vi "continue frame scan.vi"(7 "Max queue size":i32, 8 "Error in":errorcluster, 10 "Scan Status in":enum16{"Start", "Continue Scan", "Finish Scan"}(ring), 11 "Scan Type [in":T1) -> (0 "Error Out":errorcluster)   [LabVIEW 2018]
uses:
  Controls/ScanType.ctl
  Controls/QueueNames.ctl
  Controls/MessagePacket.ctl
  Controls/Queue Manager Actions.ctl
  Controls/FGV Actions.ctl
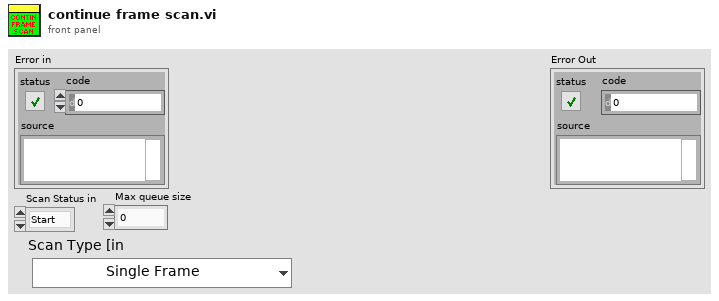
[diagram p1: front panel]
types:
  T1 = typedef "ScanType.ctl" = enum16{"Single Frame", "Continuous Frame", "ROI Line", "Vibratome", "Mosaic", "Mosaic + Slice"}
  T2 = typedef "Queue Manager Actions.ctl" = enum16{"Init", "Enqueue", "Enqueue All", "Preview Queue", "Dequeue", "Get Status", "Flush Queue", "Flush All Queues", "Release All Queues", "Release Queue", "Enqueue at Opposite End"}
  T3 = typedef "MessagePacket.ctl" = cluster{"Message":string, "Parameter":variant}
  T4 = typedef "QueueNames.ctl" = enum16{"Main GUI", "Main Scan Processor", "Main Processing", "Main Saving", "Main Display", "Main Table Stage GUI", "Main Table Stage Proc.", "Scan Engine", "Vibratome GUI", "Vibratome Processor", "Slice Engine"}
  T5 = typedef "FGV Actions.ctl" = enum16{"Init", "Set", "Get", "Clear"}
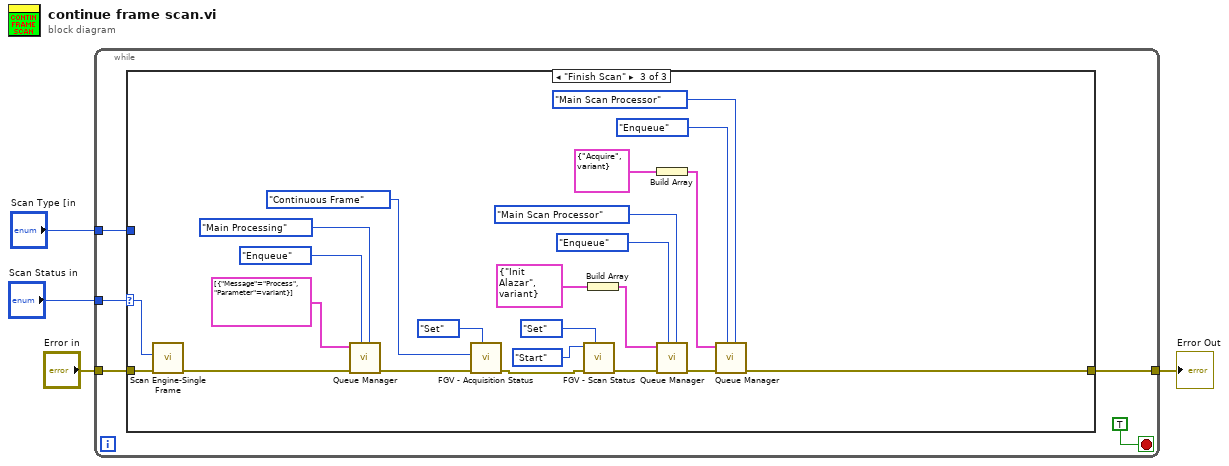
[diagram p0: block diagram]
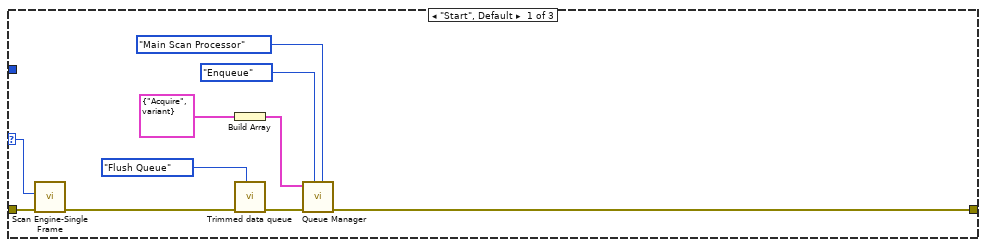
[diagram p2: hidden frame]
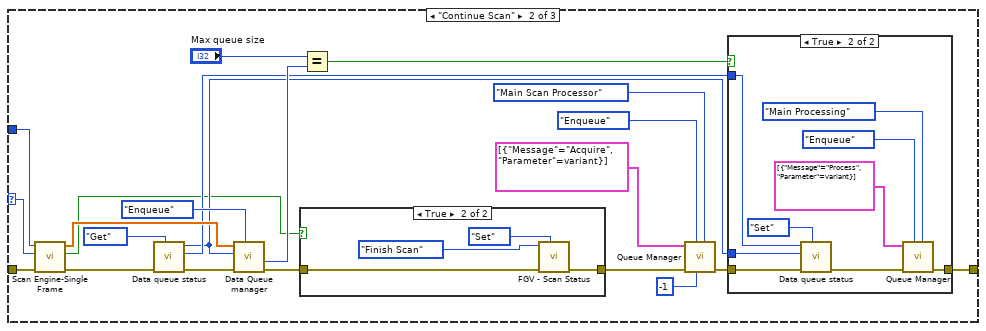
[diagram p3: hidden frame]
diagram:
  n1 = while {
    tunnel: "Scan Status in" -> [w9]
    tunnel: "Error in" -> [w8]
    tunnel: "Scan Type [in" -> [w7]
    tunnel: [w6] -> w1
    stop <- TRUE stop-if-true
    n2 = case shown="\"Finish Scan\"" w9 {
      selector: w9 -> [w18 w34 w79]
      tunnel: w8 -> [w19 w41 w78]
      tunnel: [w13 w27 w71] -> w6
      tunnel: w7 -> [_ w24 _]
      frame "Start", Default {
        n3 = call "Scan Engine-Single Frame.vi"("Error in"=w19, "Scan Status"=w18) -> ("Error Out"=w14:errorcluster)  [unwired: 7 in, 2 out]
        n4 = Build Array(T3 {"Message"="Acquire", "Parameter"=variant} ("Message Packet [In]")) -> (w15:T3[])
        n5 = call "Trimmed data queue.vi"("Action"=Queue_Manager_Actions."Flush Queue", "error in (no error)"=w14) -> ("error out"=w11:errorcluster)  [unwired: 6 in, 3 out]
        n6 = call "Queue Manager.vi"("Queue Name"=QueueNames."Main Scan Processor", "Action"=Queue_Manager_Actions."Enqueue", "Error In"=w11, "Message Packet Array"=w15) -> ("Error Out"=w13:errorcluster)  [unwired: 3 in, 4 out]
      }
      frame "Continue Scan" {
        n7 = call "Scan Engine-Single Frame.vi"("Error in"=w41, "Scan Status"=w34, "Scan Type in"=w24) -> ("Error Out"=w33:errorcluster, "task done?"=w21:bool, "data out"=w35:sgl[])  [unwired: 6 in]
        n8 = call "Data queue status.vi"("action"=enum16{"Init", "Get", "Set"}."Get", "error in"=w33) -> ("error out"=w32:errorcluster, "dequeue channel"=w26:enum16{"1", "2"}, "enqueue channel"=w25:enum16{"1", "2"})  [unwired: 7 in]
        n9 = call "Data Queue manager.vi"("Action"=Queue_Manager_Actions."Enqueue", "error in"=w32, "enqueue channel"=w25, "Buffer"=w35) -> ("error out"=w23:errorcluster, "# elements in queue"=w30:i32)  [unwired: 4 in, 2 out]
        n10 = case shown="True" w21 {
          tunnel: w23 -> [w42 w45]
          tunnel: [w42 w44] -> w22
          frame False {
          }
          frame True {
            n11 = call "FGV - Scan Status.vi"("Actions"=FGV_Actions."Set", "Error In"=w45, "Scan Status in"=enum16{"Start", "Continue Scan", "Finish Scan"}."Finish Scan") -> ("Error Out"=w44:errorcluster)  [unwired: 6 in, 2 out]
          }
        }
        n12 = Equal?(x="Max queue size", y=w30) -> (x = y?=w29:bool)
        n13 = call "Queue Manager.vi"("Queue Name"=QueueNames."Main Scan Processor", "timeout in ms (-1)"=-1, "Action"=Queue_Manager_Actions."Enqueue", "Error In"=w22, "Message Packet Array"=T3[] [{"Message"="Acquire", "Parameter"=variant}] ("Message Packet [In]")) -> ("Error Out"=w28:errorcluster)  [unwired: 2 in, 4 out]
        n14 = case shown="True" w29 {
          tunnel: [w47 w51] -> w27
          tunnel: w28 -> [w47 w49]
          tunnel: w26 -> [_ w55]
          tunnel: w25 -> [_ w54]
          frame False {
          }
          frame True {
            n15 = call "Data queue status.vi"("action"=enum16{"Init", "Get", "Set"}."Set", "error in"=w49, "dequeue channel"=w54, "enqueue channel"=w55) -> ("error out"=w48:errorcluster)  [unwired: 5 in, 2 out]
            n16 = call "Queue Manager.vi"("Queue Name"=QueueNames."Main Processing", "Action"=Queue_Manager_Actions."Enqueue", "Error In"=w48, "Message Packet Array"=T3[] [{"Message"="Process", "Parameter"=variant}]) -> ("Error Out"=w51:errorcluster)  [unwired: 3 in, 4 out]
          }
        }
      }
      frame "Finish Scan" {
        n17 = call "Scan Engine-Single Frame.vi"("Error in"=w78, "Scan Status"=w79) -> ("Error Out"=w61:errorcluster)  [unwired: 7 in, 2 out]
        n18 = call "Queue Manager.vi"("Queue Name"=QueueNames."Main Processing", "Action"=Queue_Manager_Actions."Enqueue", "Error In"=w61, "Message Packet Array"=T3[] [{"Message"="Process", "Parameter"=variant}]) -> ("Error Out"=w60:errorcluster)  [unwired: 3 in, 4 out]
        n19 = call "FGV - Acquisition Status.vi"("Actions"=FGV_Actions."Set", "Error In"=w60, "Scan Type [In]"=ScanType."Continuous Frame") -> ("Error Out"=w59:errorcluster)  [unwired: 6 in, 2 out]
        n20 = call "FGV - Scan Status.vi"("Actions"=FGV_Actions."Set", "Error In"=w59, "Scan Status in"=enum16{"Start", "Continue Scan", "Finish Scan"}."Start") -> ("Error Out"=w66:errorcluster)  [unwired: 6 in, 2 out]
        n21 = Build Array(T3 {"Message"="Init Alazar", "Parameter"=variant} ("Message Packet [In]")) -> (w67:T3[])
        n22 = Build Array(T3 {"Message"="Acquire", "Parameter"=variant} ("Message Packet [In]")) -> (w74:T3[])
        n23 = call "Queue Manager.vi"("Queue Name"=QueueNames."Main Scan Processor", "Action"=Queue_Manager_Actions."Enqueue", "Error In"=w66, "Message Packet Array"=w67) -> ("Error Out"=w65:errorcluster)  [unwired: 3 in, 4 out]
        n24 = call "Queue Manager.vi"("Queue Name"=QueueNames."Main Scan Processor", "Action"=Queue_Manager_Actions."Enqueue", "Error In"=w65, "Message Packet Array"=w74) -> ("Error Out"=w71:errorcluster)  [unwired: 3 in, 4 out]
      }
    }
  }
  "Error Out" <- w1
